vi "Experiment 5.vi"() -> ()   [LabVIEW 2026]
doc: "Experiment 5"
uses:
  <vilib>/Analysis/baseanly.llb/Mean (DBL).vi
  <vilib>/Analysis/NI_AALBase.lvlib
panel:
  out "Execution Time - Per Call (us)":dbl format="%.6f"
  out "Execution Time - 1M Calls (seconds)":dbl format="%.6f"
  out "Output":dbl[](array[numeric]) format="%.3f"
  # "Experiment 5"
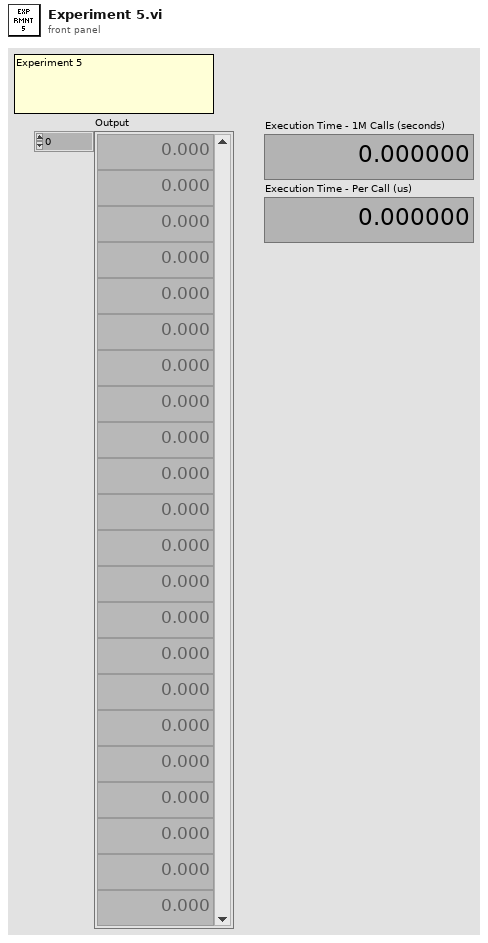
[diagram p1: front panel]
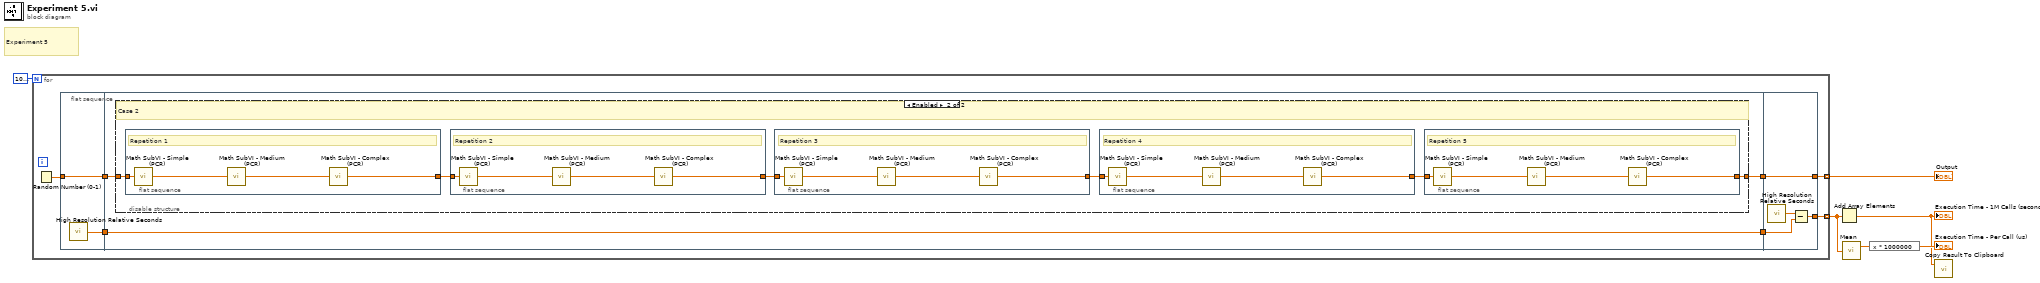
[diagram p0: block diagram]
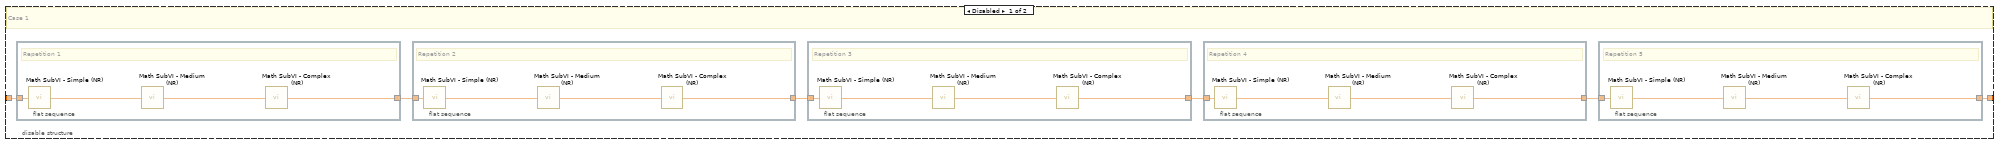
[diagram p2: hidden frame]
diagram:
  # "Experiment 5"
  n1 = for {
    N: 1000000 -> [_]
    tunnel: [w13] -> w6 mode=indexing
    tunnel: [w7] -> w4 mode=indexing
    n2 = Random Number (0-1)() -> (number: 0 to 1=w12:dbl)
    n3 = flat-sequence {
      tunnel: w12 -> [w15]
      tunnel: [w15] -> w11
      tunnel: [w14] -> w8
      tunnel: w11 -> [w16]
      tunnel: [w17] -> w10
      tunnel: [w18] -> w9
      tunnel: w8 -> [w18]
      tunnel: [w74] -> w13
      tunnel: w10 -> [w74]
      tunnel: w9 -> [w72]
      tunnel: [w71] -> w7
      frame #0 {
        n4 = call <vilib>:"High Resolution Relative Seconds.vi"() -> ("relative seconds"=w14:dbl)
      }
      frame #1 {
        n5 = disable-structure shown="Enabled" {
          disable-tunnel: [w19 w45] -> w17
          disable-tunnel: w16 -> [w24 w50]
          frame Disabled {
            # "Case 1"
            n6 = flat-sequence {
              tunnel: w24 -> [w43]
              tunnel: [w41] -> w23
              frame #0 {
                # "Repetition 1"
                n7 = call "Math SubVI - Simple (NR).vi"("Input"=w43) -> ("Output"=w44:dbl)
                n8 = call "Math SubVI - Medium (NR).vi"("Input"=w44) -> ("Output"=w42:dbl)
                n9 = call "Math SubVI - Complex (NR).vi"("Input"=w42) -> ("Output"=w41:dbl)
              }
            }
            n10 = flat-sequence {
              tunnel: w23 -> [w39]
              tunnel: [w37] -> w22
              frame #0 {
                # "Repetition 2"
                n11 = call "Math SubVI - Simple (NR).vi"("Input"=w39) -> ("Output"=w40:dbl)
                n12 = call "Math SubVI - Medium (NR).vi"("Input"=w40) -> ("Output"=w38:dbl)
                n13 = call "Math SubVI - Complex (NR).vi"("Input"=w38) -> ("Output"=w37:dbl)
              }
            }
            n14 = flat-sequence {
              tunnel: w22 -> [w35]
              tunnel: [w33] -> w21
              frame #0 {
                # "Repetition 3"
                n15 = call "Math SubVI - Simple (NR).vi"("Input"=w35) -> ("Output"=w36:dbl)
                n16 = call "Math SubVI - Medium (NR).vi"("Input"=w36) -> ("Output"=w34:dbl)
                n17 = call "Math SubVI - Complex (NR).vi"("Input"=w34) -> ("Output"=w33:dbl)
              }
            }
            n18 = flat-sequence {
              tunnel: w21 -> [w31]
              tunnel: [w29] -> w20
              frame #0 {
                # "Repetition 4"
                n19 = call "Math SubVI - Simple (NR).vi"("Input"=w31) -> ("Output"=w32:dbl)
                n20 = call "Math SubVI - Medium (NR).vi"("Input"=w32) -> ("Output"=w30:dbl)
                n21 = call "Math SubVI - Complex (NR).vi"("Input"=w30) -> ("Output"=w29:dbl)
              }
            }
            n22 = flat-sequence {
              tunnel: w20 -> [w27]
              tunnel: [w25] -> w19
              frame #0 {
                # "Repetition 5"
                n23 = call "Math SubVI - Simple (NR).vi"("Input"=w27) -> ("Output"=w28:dbl)
                n24 = call "Math SubVI - Medium (NR).vi"("Input"=w28) -> ("Output"=w26:dbl)
                n25 = call "Math SubVI - Complex (NR).vi"("Input"=w26) -> ("Output"=w25:dbl)
              }
            }
          }
          frame Enabled {
            # "Case 2"
            n26 = flat-sequence {
              tunnel: w50 -> [w69]
              tunnel: [w67] -> w49
              frame #0 {
                # "Repetition 1"
                n27 = call "Math SubVI - Simple (PCR).vi"("Input"=w69) -> ("Output"=w70:dbl)
                n28 = call "Math SubVI - Medium (PCR).vi"("Input"=w70) -> ("Output"=w68:dbl)
                n29 = call "Math SubVI - Complex (PCR).vi"("Input"=w68) -> ("Output"=w67:dbl)
              }
            }
            n30 = flat-sequence {
              tunnel: w49 -> [w65]
              tunnel: [w63] -> w48
              frame #0 {
                # "Repetition 2"
                n31 = call "Math SubVI - Simple (PCR).vi"("Input"=w65) -> ("Output"=w66:dbl)
                n32 = call "Math SubVI - Medium (PCR).vi"("Input"=w66) -> ("Output"=w64:dbl)
                n33 = call "Math SubVI - Complex (PCR).vi"("Input"=w64) -> ("Output"=w63:dbl)
              }
            }
            n34 = flat-sequence {
              tunnel: w48 -> [w61]
              tunnel: [w59] -> w47
              frame #0 {
                # "Repetition 3"
                n35 = call "Math SubVI - Simple (PCR).vi"("Input"=w61) -> ("Output"=w62:dbl)
                n36 = call "Math SubVI - Medium (PCR).vi"("Input"=w62) -> ("Output"=w60:dbl)
                n37 = call "Math SubVI - Complex (PCR).vi"("Input"=w60) -> ("Output"=w59:dbl)
              }
            }
            n38 = flat-sequence {
              tunnel: w47 -> [w57]
              tunnel: [w55] -> w46
              frame #0 {
                # "Repetition 4"
                n39 = call "Math SubVI - Simple (PCR).vi"("Input"=w57) -> ("Output"=w58:dbl)
                n40 = call "Math SubVI - Medium (PCR).vi"("Input"=w58) -> ("Output"=w56:dbl)
                n41 = call "Math SubVI - Complex (PCR).vi"("Input"=w56) -> ("Output"=w55:dbl)
              }
            }
            n42 = flat-sequence {
              tunnel: w46 -> [w53]
              tunnel: [w51] -> w45
              frame #0 {
                # "Repetition 5"
                n43 = call "Math SubVI - Simple (PCR).vi"("Input"=w53) -> ("Output"=w54:dbl)
                n44 = call "Math SubVI - Medium (PCR).vi"("Input"=w54) -> ("Output"=w52:dbl)
                n45 = call "Math SubVI - Complex (PCR).vi"("Input"=w52) -> ("Output"=w51:dbl)
              }
            }
          }
        }
      }
      frame #2 {
        n46 = call <vilib>:"High Resolution Relative Seconds.vi"() -> ("relative seconds"=w73:dbl)
        n47 = Subtract(x=w73, y=w72) -> (x-y=w71:dbl)
      }
    }
  }
  "Output" <- w6
  n48 = Add Array Elements(numeric array=w4) -> (sum=w1:dbl)
  "Execution Time - 1M Calls (seconds)" <- w1
  n49 = call-poly <vilib>:"Mean.vi"("X"=w4) -> ("mean"=w3:dbl)  [unwired: 1 out]
  n50 = expression code="x * 1000000"(w3) -> (→"Execution Time - Per Call (us)":dbl)
  n51 = call "Copy Result To Clipboard.vi"("Input"=w1) -> ()  [unwired: 1 in]
